vi "Enter_Rock_Data.vi"() -> ()   [LabVIEW 2019]
uses:
  Calibration.ctl
  <vilib>/Utility/NIReport.llb/Report Type.ctl
  <vilib>/addons/database/Connection.llb/DB Tools Open Connec (Path).vi
  <vilib>/addons/_office/word.llb/Word Find & Replace (str).vi
  <vilib>/addons/database/_DB Variant To Data/Database Variant To Data.xnode
  <vilib>/Utility/NIReport.llb/NI_report.lvclass
  <vilib>/addons/database/NI_Database_API.lvlib
  TEST.lvclass
  <vilib>/Utility/NIReport.llb/NI_ReportGenerationCore.lvlib
  <vilib>/addons/_office/NI_ReportGenerationToolkit.lvlib
  <vilib>/Utility/NIReport.llb/Word/NI_Word.lvclass
panel:
  in  "校准日期":timestamp format="%<%Y/%m/%d>T"
  in  "生产日期":timestamp format="%<%Y/%m/%d>T"
  in  "批号":string
  out "下沉位置":string[](array[string])
  out "误差%":string[](array[string])
  out "最大偏差":string[](array[string])
  out "测试力标准值":string[](array[string])
  in  "data":sgl[][](array[numeric]) format="%#.2g"
  out "初始化成功":bool
  out "error out":errorcluster
  in  "init":bool
  in  "NAME":string
  out "HS2":string[](array[string])
  out "CFXWC":string[](array[string])
  out "HAWC":string[](array[string])
  out "允许误差%":string[](array[string])
  out "试验力N(kg)":string[](array[string])
  out "执行状态":bool
  out "数据写入成功":bool
  in  "print_calibration":bool
  in  "print_data":bool
  in  "核验员":string
  in  "tsd":sgl[](array[numeric])=[1.0, 1.0, 1.0, 1.0] format="%#.2g"
  in  "停止":bool
  in  "write":bool
  in  "clear":bool
  in  "TEMP":string
  in  "TSN":string
  in  "MODE":string
  out "REP":sgl[](array[numeric]) format="%#.2g"
  out "HV":sgl[](array[numeric]) format="%#.2g"
  out "AVG":sgl[](array[numeric]) format="%#.2g"
  in  "TV":sgl[][](array[numeric]) format="%#.2g"
  in  "HS":sgl[](array[numeric])=[0.0, 0.0, 0.0, 0.0, 0.0] format="%#.2g"
  in  "HN":string[](array[string])
  out "Test":sgl[][](array[numeric]) format="%#.2g"
  in  "DIN":string
  out "Inacc":sgl[](array[numeric]) format="%#.2g"
  out "Dev":sgl[](array[numeric]) format="%#.2g"
  # "产品名称(首填)："
  # "型号："
  # "制造编号："
  # "温度："
  # "℃"
  # "试验力测试"
  # "2"
  # "3"
  # "1"
  # "±"
  # "±"
  # "±"
  # "±"
  # "硬度测试"
  # "金刚石压头编号："
  # "测试值"
  # "硬度块\n标准值"
  # "硬度块\n  编号"
  # "硬度值"
  # "重复性"
  # "平均值"
  # "1"
  # "2"
  # "4"
  # "5"
  # "3"
  # "实际误差"
  # "允许误差"
  # "实际误差"
  # "允许误差"
  # "±1.0"
  # "1.0RA"
  # "RA"
  # "±1.5"
  # "1.5RB"
  # "RB"
  # "±1.5"
  # "1.5RC"
  # "RC"
  # "±1.2"
  # "1.2RC"
  # "RC"
  # "±1.0"
  # "1.2RC"
  # "RC"
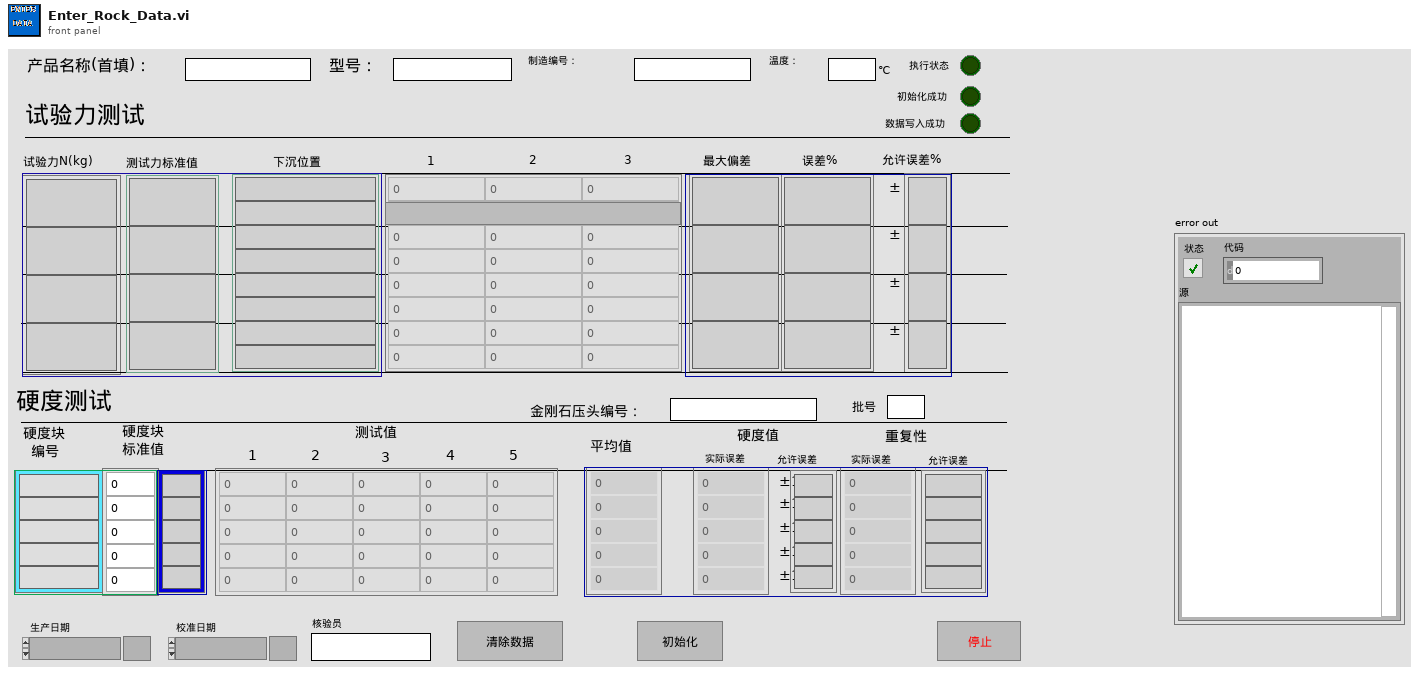
[diagram p1: front panel]
types:
  T1 = enum8{"Enabled", "Disabled", "Disabled and Grayed Out"}
  T2 = enum16{"open", "replace", "create", "open or create", "replace or create", "replace or create with confirmation"}
  T3 = typedef "TEST.lvclass/Calibration.ctl" = cluster{"NAM":string, "MODE":string, "TSN":string, "TDN":string, "DIN":string, "PROD":string, "CALD":string, "REV":string}
  T4 = typedef "NI_ReportGenerationCore.lvlib/Report Type.ctl" = enum16{"HTML", "Word", "Excel"}
  T5 = enum16{"maximized", "minimized", "normal", "no change"}
  T6 = typedef "NI_Database_API.lvlib/Conn ObjectReference.ctl" = refnum<k1>
  T7 = typedef "NI_Database_API.lvlib/DB Tools DataTypes.ctl" = enum16{"String", "Long (I32)", "Single (SGL)", "Double (DBL)", "Date/Time", "Binary"}
  T8 = cluster{"name":string, "database data type":T7, "defined size":i32}[]
  T9 = cluster{"name":string, "database data type":T7, "defined size":i32, bool}
  T10 = typedef "TEST.lvclass/Test_data.ctl" = cluster{"MODE":string, "TSN":string, "Temp":string, "Test_load_row1":T11, "Test_load_row2":T11, "Test_load_row3":T11, "Test_load_row4":T11, "DIN":string, "Hardness_test_row1":T12, "Hardness_test_row2":T12, "Hardness_test_row3":T12, "Hardness_test_row4":T12, "Hardness_test_row5":T12}
  T11 = typedef "TEST.lvclass/Test_load.ctl" = cluster{"TEST1":sgl, "TEST2":sgl, "TEST3":sgl, "DEV":sgl, "INACC":sgl}
  T12 = typedef "TEST.lvclass/Hardness_test.ctl" = cluster{"HN":string, "HS":sgl, "TV1":sgl, "TV2":sgl, "TV3":sgl, "TV4":sgl, "TV5":sgl, "AVG":sgl, "HV":sgl, "REP":sgl}
  T13 = typedef "TEST.lvclass/Cluster67.ctl" = cluster{"MOD":string, "TSN":string, "Temp":string, "TEST1":sgl, "TEST2":sgl, "TEST3":sgl, "DEV":sgl, "INACC":sgl, "TEST1":sgl, "TEST2":sgl, "TEST3":sgl, "DEV":sgl, "INACC":sgl, "TEST1":sgl, "TEST2":sgl, "TEST3":sgl, "DEV":sgl, "INACC":sgl, "TEST1":sgl, "TEST2":sgl, "TEST3":sgl, "DEV":sgl, "INACC":sgl, "DIN":string, "HN":string, "HS":sgl, "TV1":sgl, "TV2":sgl, "TV3":sgl, "TV4":sgl, "TV5":sgl, "AVG":sgl, "HV":sgl, "REP":sgl, "HN":string, "HS":sgl, "TV1":sgl, "TV2":sgl, "TV3":sgl, "TV4":sgl, "TV5":sgl, "AVG":sgl, "HV":sgl, "REP":sgl, "HN":string, "HS":sgl, "TV1":sgl, "TV2":sgl, "TV3":sgl, "TV4":sgl, "TV5":sgl, "AVG":sgl, "HV":sgl, "REP":sgl, "HN":string, "HS":sgl, "TV1":sgl, "TV2":sgl, "TV3":sgl, "TV4":sgl, "TV5":sgl, "AVG":sgl, "HV":sgl, "REP":sgl, "HN":string, "HS":sgl, "TV1":sgl, "TV2":sgl, "TV3":sgl, "TV4":sgl, "TV5":sgl, "AVG":sgl, "HV":sgl, "REP":sgl, "NAM":string, "TDN":string, "PROD":string, "CALD":string, "REV":string}
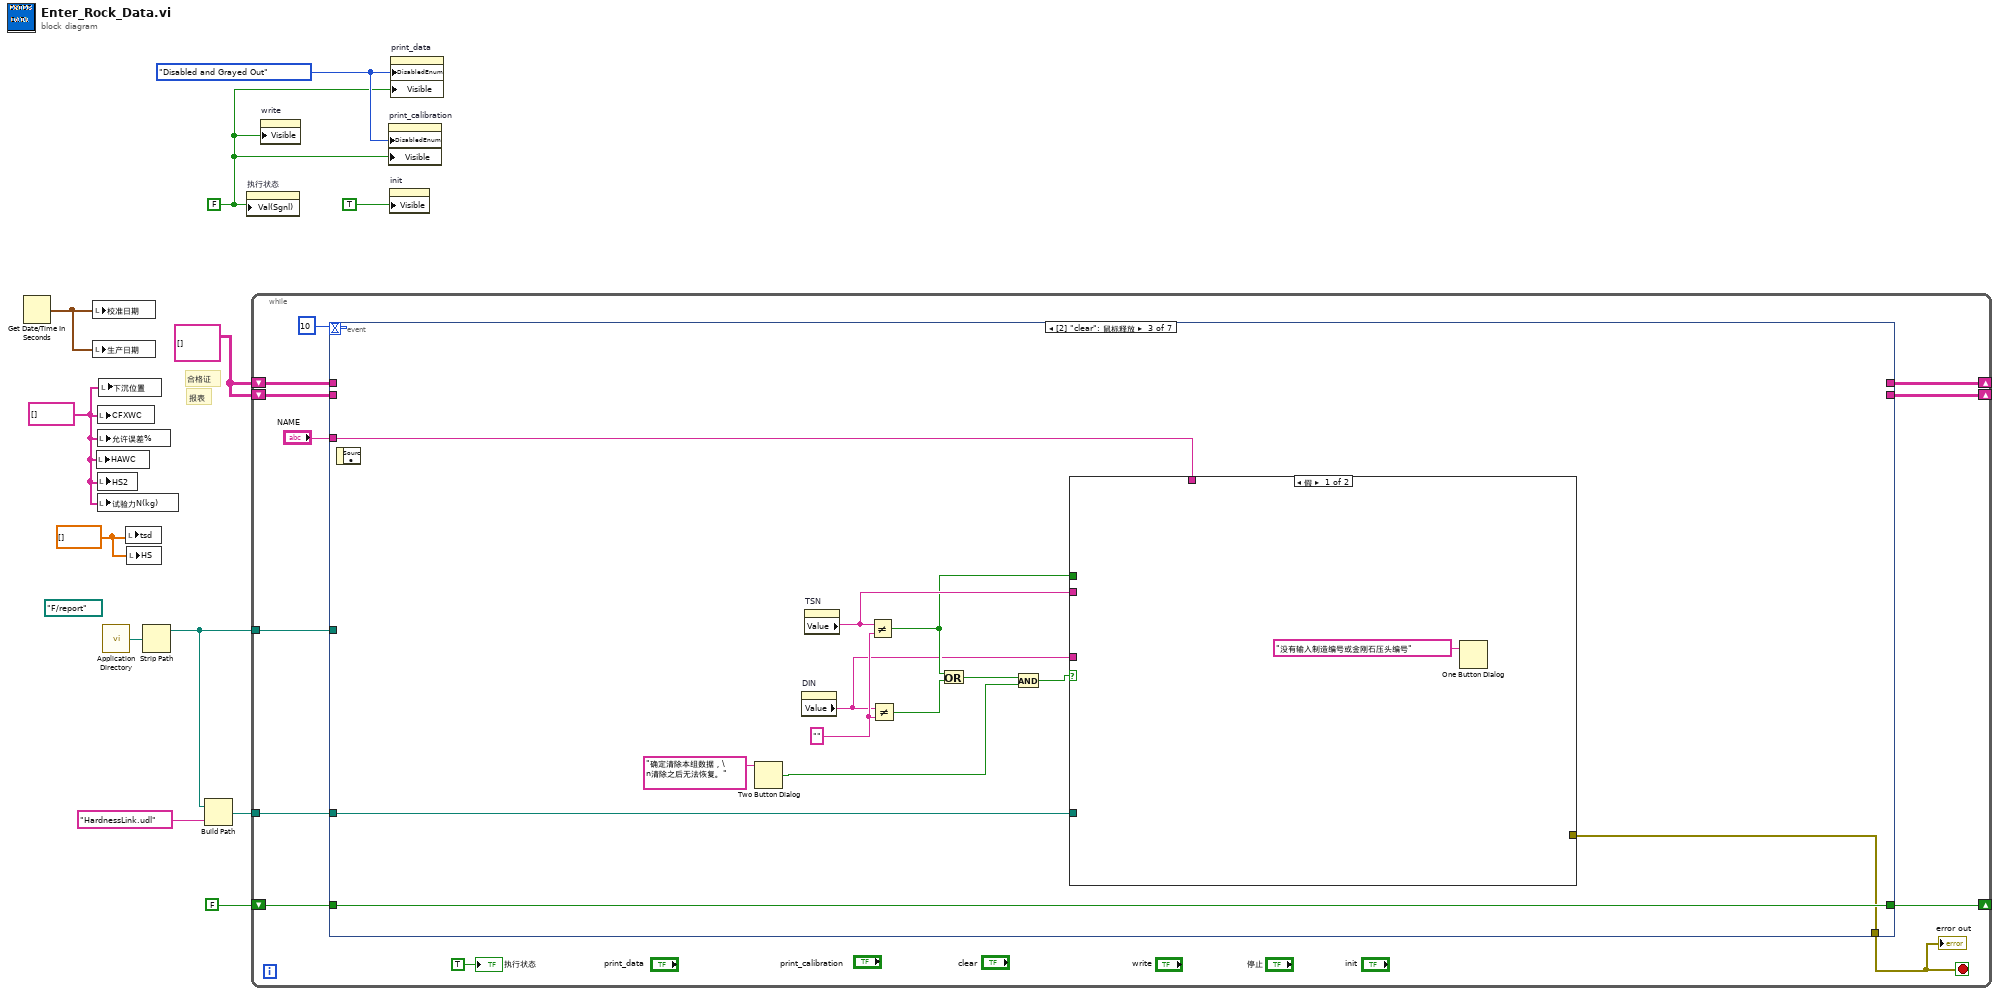
[diagram p0: block diagram]
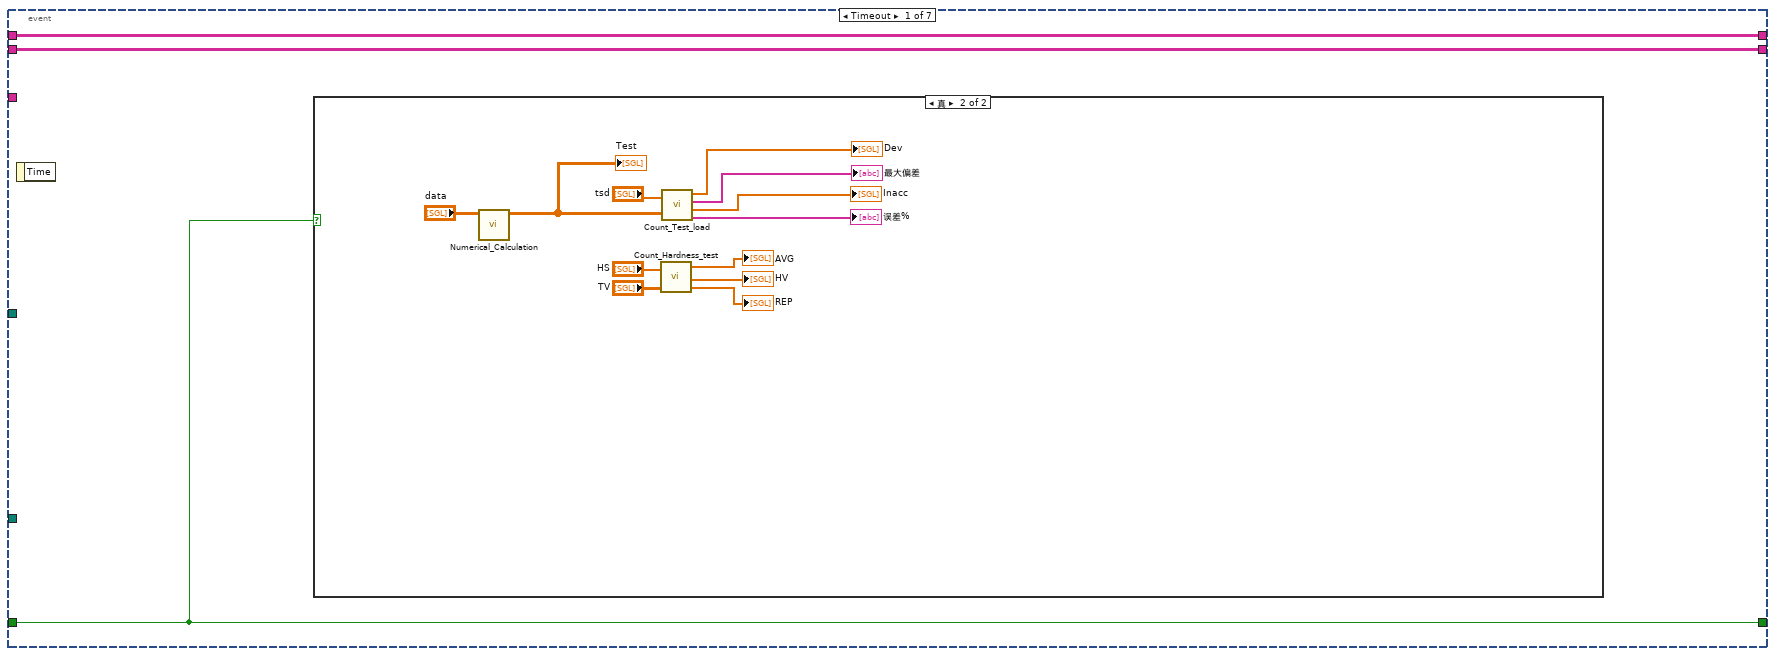
[diagram p2: hidden frame]
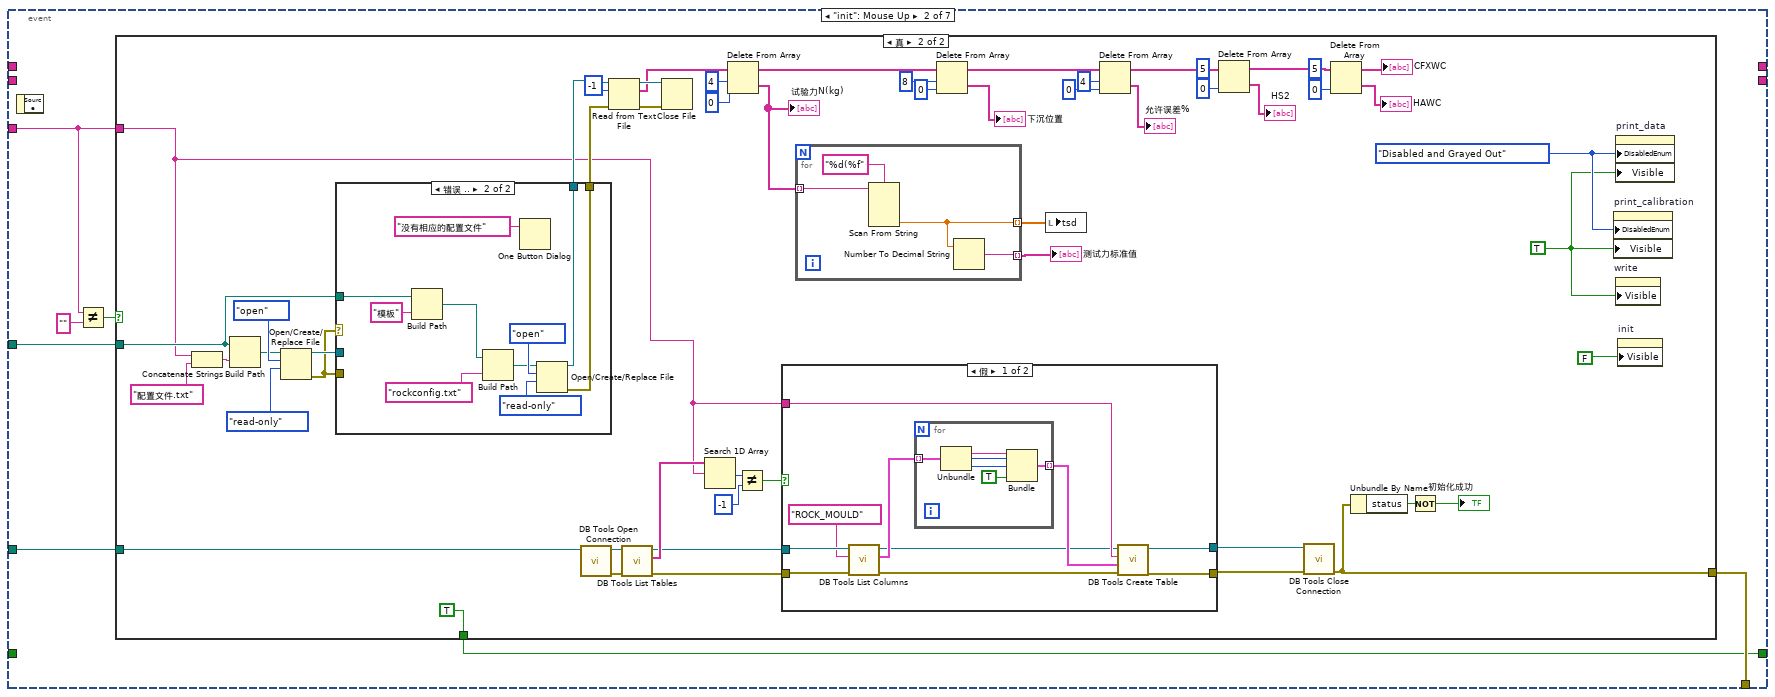
[diagram p4: hidden frame]
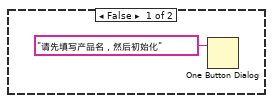
[diagram p5: hidden frame]
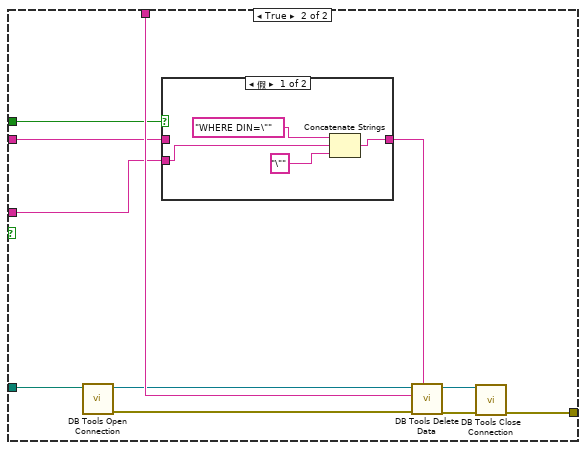
[diagram p8: hidden frame]
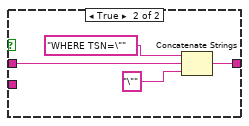
[diagram p9: hidden frame]
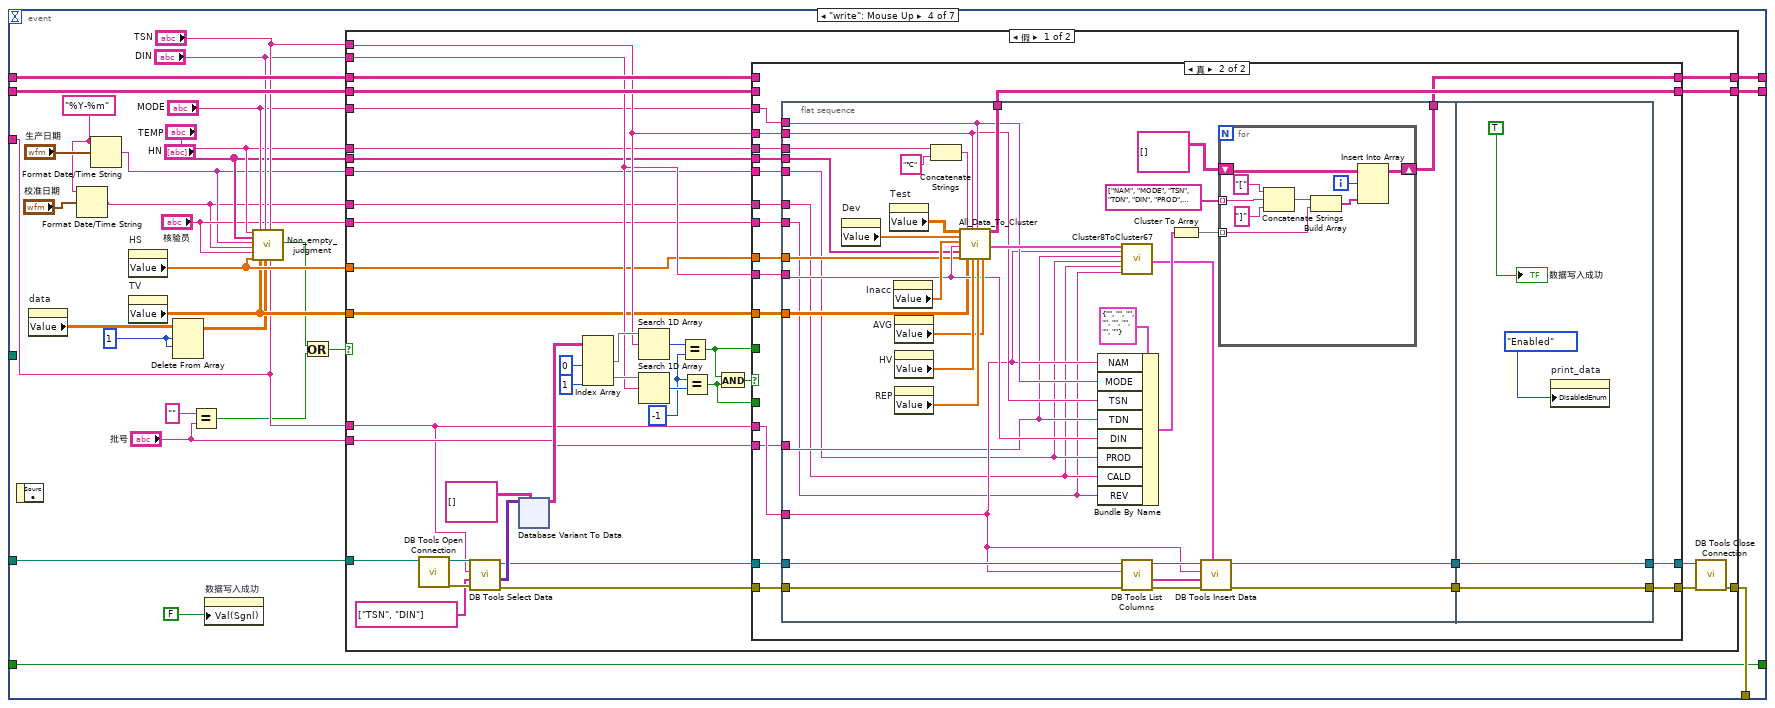
[diagram p10: hidden frame]
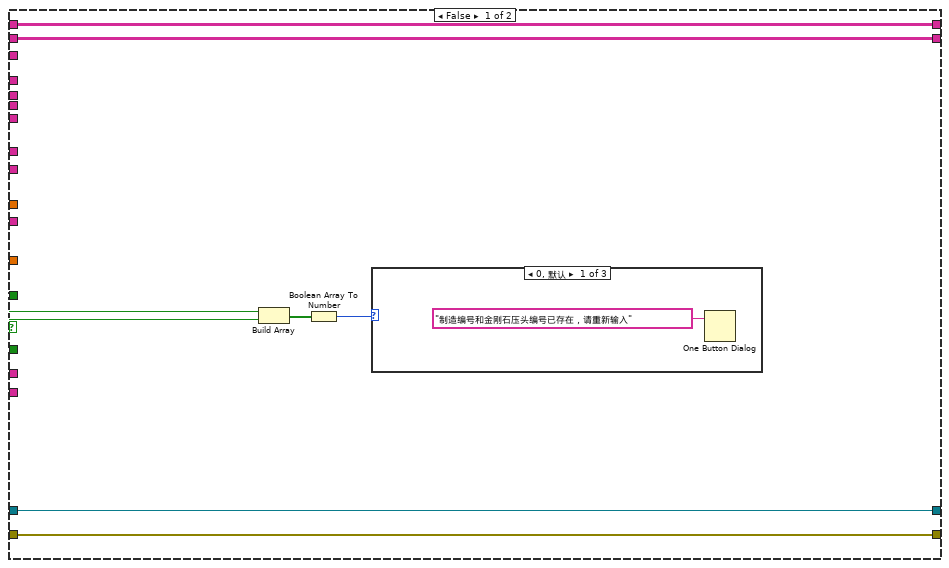
[diagram p11: hidden frame]
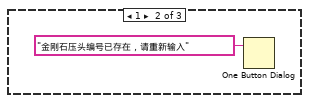
[diagram p12: hidden frame]
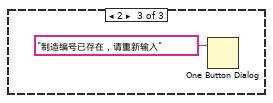
[diagram p13: hidden frame]
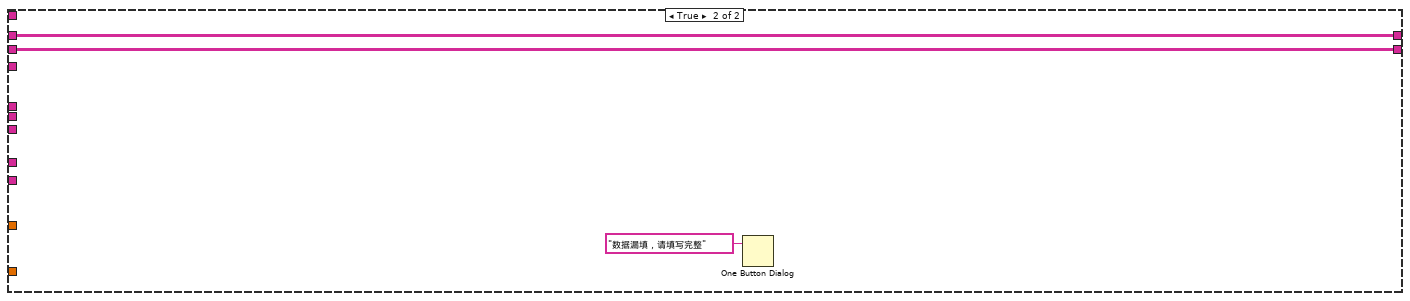
[diagram p14: hidden frame]
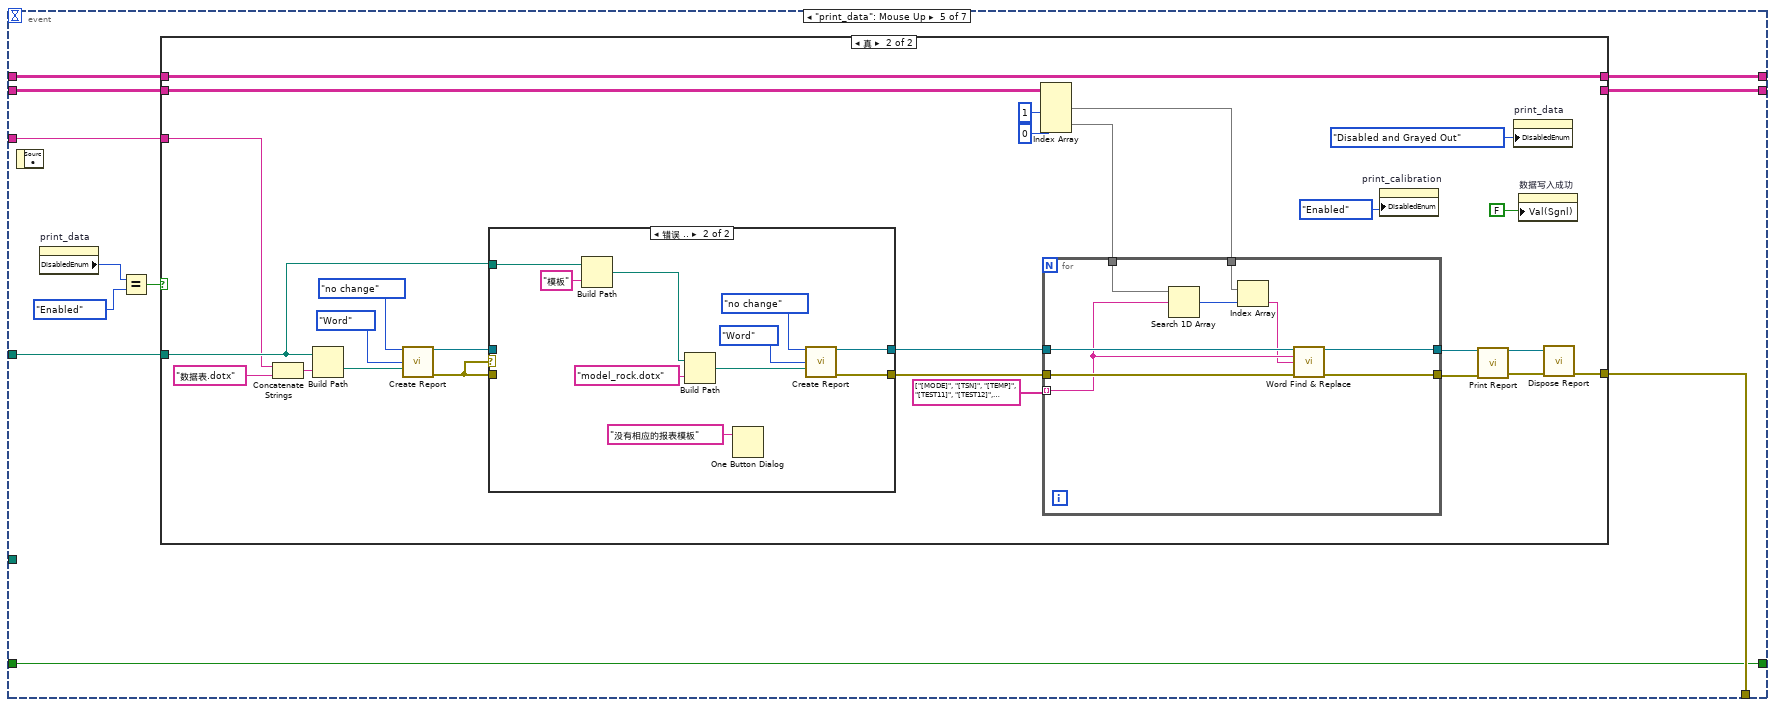
[diagram p15: hidden frame]
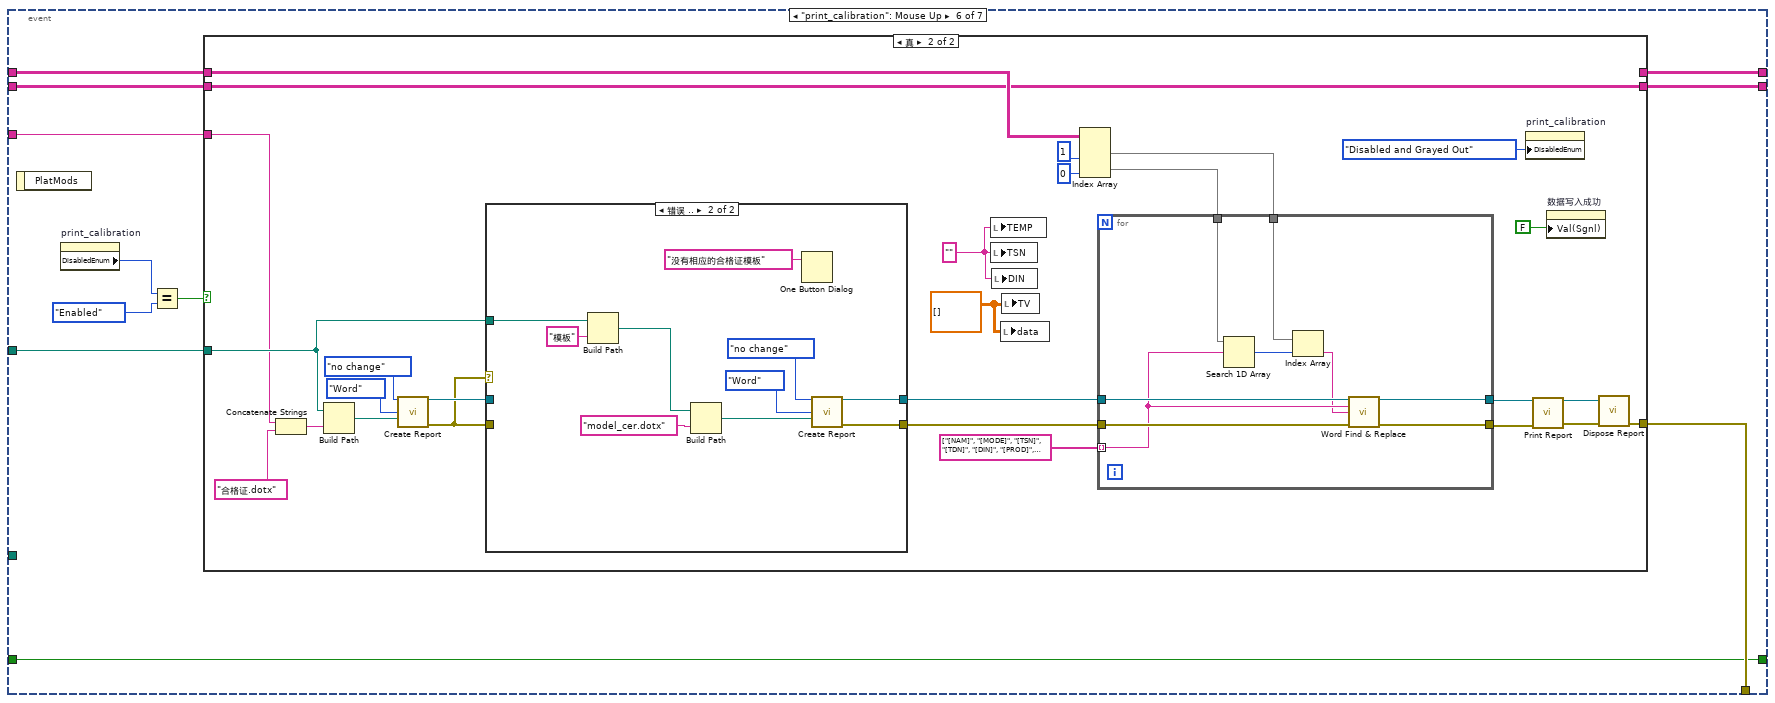
[diagram p18: hidden frame]
diagram:
  w9 = sgl[] []
  w7 = string[] []
  (unwired) path "F:/report" ("data__in")
  w8 = FALSE
  w12 = T1."Disabled and Grayed Out" ("禁用")
  w11 = string[][] []
  # "报表"
  # "合格证"
  n1 = Get Date/Time In Seconds() -> (seconds since 1Jan1904=w1:timestamp)
  n2 = local write "校准日期"(w1) -> ()
  n3 = local write "生产日期"(w1) -> ()
  n4 = local write "HAWC"(w7) -> ()
  n5 = local write "CFXWC"(w7) -> ()
  n6 = local write "允许误差%"(w7) -> ()
  n7 = local write "HS2"(w7) -> ()
  n8 = local write "试验力N(kg)"(w7) -> ()
  n9 = local write "下沉位置"(w7) -> ()
  n10 = call <vilib>:"Application Directory.vi"() -> ("Application Directory"=w5:path)
  n11 = local write "tsd"(w9) -> ()
  n12 = local write "HS"(w9) -> ()
  n13 = Strip Path(path=w5) -> (stripped path=w2:path)  [unwired: 1 out]
  n14 = Build Path(base path=w2, name or relative path="HardnessLink.udl" ("名称或相对路径")) -> (appended path=w3:path)
  n15 = property on="执行状态" class="Bool (严格)"("Val(Sgnl)"=w8) -> ()  [unwired: 2 in, 2 out]
  n16 = while {
    shift-right: [w23] -> _
    shift-left: w11 -> [w22]
    shift-right: [w20] -> _
    shift-left: w11 -> [w19]
    tunnel: w2 -> [w14]
    shift-right: [w16] -> _
    shift-left: FALSE -> [w15]
    tunnel: w3 -> [w13]
    stop <- w17 stop-if-true
    n17 = event shown="[2] \"clear\": 鼠标释放" {
      selector: _ -> [_ _ _ _ _ _ _]
      dyn-events: _ -> [_ _ _ _ _ _ _]
      timeout: 10 -> [_ _ _ _ _ _ _]
      tunnel: [_ w45 w146 w195 w375 w435 errorcluster {"status"=TRUE, "code"=0, "source"=""} ("error out")] -> w17
      tunnel: [w27 _ _ w199 w368 w430 _] -> w23
      tunnel: w22 -> [w27 _ _ w196 w371 w429 _]
      tunnel: [w26 _ _ w198 w370 w428 _] -> w20
      tunnel: w19 -> [w26 _ _ w197 w369 w431 _]
      tunnel: "NAME" -> [_ w44 w147 w186 w373 w432 _]
      tunnel: w14 -> [_ w46 _ _ w374 w434 _]
      tunnel: [w25 w41 w149 w185 w372 w433 FALSE] -> w16
      tunnel: w15 -> [w25 _ w149 w185 w372 w433 _]
      tunnel: w13 -> [_ w40 w148 w179 _ _ _]
      event Timeout {
        n18 = event-data() -> ()  [unwired: 1 in, 1 out]
        n19 = case shown="真" w25 {
          frame False {
          }
          frame True {
            n20 = call "Numerical_Calculation.vi"("Nums"="data") -> ("Calculation"=w30:sgl[][])  [unwired: 10 in]
            "Test" <- w30
            n21 = call "Count_Hardness_test.vi"("HS"="HS", "TV"="TV") -> ("AVG"=→"AVG":sgl[], "HV"=→"HV":sgl[], "REP"=→"REP":sgl[])
            n22 = call "Count_Test_load.vi"("tsd"="tsd", "Test"=w30) -> ("dev"=→"Dev":sgl[], "devs"=→"最大偏差":string[], "inacc"=→"Inacc":sgl[], "inaccs"=→"误差%":string[])
          }
        }
      }
      event "init": Mouse Up {
        n23 = event-data() -> ()  [unwired: 1 in, 1 out]
        n24 = Not Equal?(x=w44, y="" ("NAME")) -> (x != y?=w42:bool)
        n25 = case shown="真" w42 {
          tunnel: w46 -> [_ w65]
          tunnel: [_ w64] -> w45
          tunnel: w44 -> [_ w48]
          tunnel: [_ TRUE] -> w41
          tunnel: w40 -> [_ w49]
          frame False {
            n26 = One Button Dialog(message="请先填写产品名，然后初始化" ("消息")) -> ()  [unwired: 1 in, 1 out]
          }
          frame True {
            w91 = T1."Disabled and Grayed Out" ("禁用")
            w90 = TRUE ("可见")
            n27 = Concatenate Strings(w48, "配置文件.txt" ("名称或相对路径")) -> (w70:string)
            n28 = Build Path(base path=w65, name or relative path=w70) -> (appended path=w84:path)
            n29 = Open/Create/Replace File(file path (use dialog)=w84, operation (0:open)=T2."open" ("操作(0:open)"), access (0:read/write)=enum16{"read/write", "read-only", "write-only"}."read-only" ("权限(0:read/write)")) -> (refnum out=w68:refnum<file>, error out=w66:errorcluster)  [unwired: 3 in, 1 out]
            n30 = case shown="错误 .." w66 {
              tunnel: [w108 w118] -> w69
              tunnel: w68 -> [w108 _]
              tunnel: [w107 w117] -> w67
              tunnel: w66 -> [w107 _]
              tunnel: w65 -> [_ w112]
              frame No Error {
              }
              frame Error {
                n31 = Build Path(base path=w112, name or relative path="模板" ("名称或相对路径")) -> (appended path=w110:path)
                n32 = Build Path(base path=w110, name or relative path="rockconfig.txt") -> (appended path=w114:path)
                n33 = One Button Dialog(message="没有相应的配置文件" ("消息")) -> ()  [unwired: 1 in, 1 out]
                n34 = Open/Create/Replace File(file path (use dialog)=w114, operation (0:open)=T2."open" ("操作(0:open)"), access (0:read/write)=enum16{"read/write", "read-only", "write-only"}."read-only" ("权限(0:read/write)")) -> (refnum out=w118:refnum<file>, error out=w117:errorcluster)  [unwired: 3 in, 1 out]
              }
            }
            n35 = call-poly <vilib>:"DB Tools Open Connection.vi"("connection information"=w49) -> ("error out"=w101:errorcluster, "connection reference"=w102:T6)  [unwired: 7 in]
            n36 = Read from Text File(file (use dialog)=w69, count=-1 ("计数"), error in=w67) -> (refnum out=w86:refnum<file>, text=w83:string[], error out=w87:errorcluster)  [unwired: 1 in, 1 out]
            n37 = call <vilib>:"DB Tools List Tables.vi"("error in (no error)"=w101, "connection reference"=w102) -> ("error out"=w95:errorcluster, "tables"=w100:string[], "connection reference out"=w96:T6)  [unwired: 3 in]
            n38 = Close File(refnum=w86, error in=w87) -> ()  [unwired: 2 out]
            n39 = Search 1D Array(1D array=w100, element=w48) -> (index of element=w99:i32)  [unwired: 1 in]
            n40 = Delete From Array(array=w83, length=4 ("长度"), index=0 ("索引")) -> (deleted portion=w60:string[], array with subset deleted=w80:string[])
            "试验力N(kg)" <- w60
            n41 = Not Equal?(x=w99, y=-1) -> (x != y?=w97:bool)
            n42 = case shown="假" w97 {
              tunnel: [w120 w136] -> w93
              tunnel: w96 -> [w128 w136]
              tunnel: w95 -> [w127 w135]
              tunnel: [w119 w135] -> w94
              tunnel: w48 -> [w123 _]
              frame False {
                n43 = call <vilib>:"DB Tools List Columns.vi"("error in (no error)"=w127, "table"="ROCK_MOULD", "connection reference"=w128) -> ("error out"=w121:errorcluster, "column information"=w125:T8, "connection reference out"=w122:T6)  [unwired: 1 in, 1 out]
                n44 = for {
                  tunnel: w125 -> [w134] mode=indexing
                  tunnel: [w129] -> w124 mode=indexing
                  n45 = Unbundle(w134) -> ("name"=w133:string, "database data type"=w132:T7, "defined size"=w131:i32)
                  n46 = Bundle("name"=w133, "database data type"=w132, "defined size"=w131, TRUE) -> (w129:T9)  [unwired: 1 in]
                }
                n47 = call <vilib>:"DB Tools Create Table.vi"("error in (no error)"=w121, "column information"=w124, "table"=w123, "connection reference"=w122) -> ("error out"=w119:errorcluster, "connection reference out"=w120:T6)  [unwired: 4 in]
              }
              frame True {
              }
            }
            n48 = for {
              tunnel: w60 -> [w105] mode=indexing
              tunnel: [w104] -> w61 mode=indexing
              tunnel: [w103] -> w55 mode=indexing
              n49 = Scan From String(format string="%d(%f" ("格式字符串"), input string=w105) -> (output 2=w104:dbl)  [unwired: 5 in, 3 out]
              n50 = Number To Decimal String(number=w104) -> (decimal integer string=w103:string)  [unwired: 1 in]
            }
            "测试力标准值" <- w55
            n51 = Delete From Array(array=w80, length=8 ("长度"), index=0 ("索引")) -> (deleted portion=→"下沉位置":string[], array with subset deleted=w54:string[])
            n52 = local write "tsd"(w61) -> ()
            n53 = Delete From Array(array=w54, length=4 ("长度"), index=0 ("索引")) -> (deleted portion=→"允许误差%":string[], array with subset deleted=w77:string[])
            n54 = Delete From Array(array=w77, length=5 ("长度"), index=0 ("索引")) -> (deleted portion=→"HS2":string[], array with subset deleted=w74:string[])
            n55 = call <vilib>:"DB Tools Close Connection.vi"("error in (no error)"=w94, "connection reference"=w93) -> ("error out"=w64:errorcluster)  [unwired: 5 in]
            n56 = Delete From Array(array=w74, length=5 ("长度"), index=0 ("索引")) -> (deleted portion=→"HAWC":string[], array with subset deleted=→"CFXWC":string[])
            n57 = Unbundle By Name(w64) -> ("status"=w63:bool)
            n58 = Not(x=w63) -> (.not. x?=→"初始化成功":bool)
            n59 = property on="print_calibration" class="Bool (严格)"("DisabledEnum"=w91, "Visible"=w90) -> ()  [unwired: 2 in, 2 out]
            n60 = property on="print_data" class="Bool (严格)"("DisabledEnum"=w91, "Visible"=w90) -> ()  [unwired: 2 in, 2 out]
            n61 = property on="write" class="Bool (严格)"("Visible"=w90) -> ()  [unwired: 2 in, 2 out]
            n62 = property on="init" class="Bool (严格)"("Visible"=FALSE ("可见")) -> ()  [unwired: 2 in, 2 out]
          }
        }
      }
      event "clear": Mouse Up {
        w145 = ""
        n63 = event-data() -> ()  [unwired: 1 in, 1 out]
        n64 = Two Button Dialog(message="确定清除本组数据，\n清除之后无法恢复。" ("消息")) -> (T button?=w138:bool)  [unwired: 2 in]
        n65 = property on="DIN" class="Str"() -> ("Value"=w141:string)  [unwired: 2 in, 2 out]
        n66 = property on="TSN" class="Str"() -> ("Value"=w143:string)  [unwired: 2 in, 2 out]
        n67 = Not Equal?(x=w143, y=w145) -> (x != y?=w142:bool)
        n68 = Not Equal?(x=w141, y=w145) -> (x != y?=w144:bool)
        n69 = Or(x=w142, y=w144) -> (x .or. y?=w139:bool)
        n70 = And(x=w139, y=w138) -> (x .and. y?=w137:bool)
        n71 = case shown="假" w137 {
          tunnel: w148 -> [_ w161]
          tunnel: w147 -> [_ w160]
          tunnel: [_ w159] -> w146
          tunnel: w143 -> [_ w153]
          tunnel: w142 -> [_ w152]
          tunnel: w141 -> [_ w151]
          frame False {
            n72 = One Button Dialog(message="没有输入制造编号或金刚石压头编号" ("消息")) -> ()  [unwired: 1 in, 1 out]
          }
          frame True {
            n73 = call-poly <vilib>:"DB Tools Open Connection.vi"("connection information"=w161) -> ("error out"=w157:errorcluster, "connection reference"=w158:T6)  [unwired: 7 in]
            n74 = case shown="假" w152 {
              tunnel: [w163 w167] -> w154
              tunnel: w153 -> [_ w166]
              tunnel: w151 -> [w162 _]
              frame False {
                n75 = Concatenate Strings("WHERE DIN=\"", w162, "\"" ("字符串")) -> (w163:string)
              }
              frame True {
                n76 = Concatenate Strings("WHERE TSN=\"", w166, "\"" ("字符串")) -> (w167:string)
              }
            }
            n77 = call <vilib>:"DB Tools Delete Data.vi"("condition"=w154, "error in (no error)"=w157, "table"=w160, "connection reference"=w158) -> ("error out"=w156:errorcluster, "connection reference out"=w155:T6)  [unwired: 6 in]
            n78 = call <vilib>:"DB Tools Close Connection.vi"("error in (no error)"=w156, "connection reference"=w155) -> ("error out"=w159:errorcluster)  [unwired: 5 in]
          }
        }
      }
      event "write": Mouse Up {
        w171 = 1 ("长度")
        w175 = "%Y-%m" ("时间格式字符串(%c)")
        n79 = event-data() -> ()  [unwired: 1 in, 1 out]
        n80 = property on="data" class="Arr (严格)"() -> ("Value"=w173:sgl[][])  [unwired: 2 in, 2 out]
        n81 = Format Date/Time String(time format string (%c)=w175, seconds (now)="校准日期") -> (date/time string=w174:string)  [unwired: 1 in]
        n82 = Format Date/Time String(time format string (%c)=w175, seconds (now)="生产日期") -> (date/time string=w177:string)  [unwired: 1 in]
        n83 = property on="HS" class="Arr (严格)"() -> ("Value"=w188:sgl[])  [unwired: 2 in, 2 out]
        n84 = property on="TV" class="Arr (严格)"() -> ("Value"=w187:sgl[][])  [unwired: 2 in, 2 out]
        n85 = Delete From Array(array=w173, length=w171, index (row)=w171) -> (array with subset deleted=w172:sgl[][])  [unwired: 1 in, 1 out]
        n86 = Equal?(x="", y="批号") -> (x = y?=w180:bool)
        n87 = property on="数据写入成功" class="Bool (严格)"("Val(Sgnl)"=FALSE) -> ()  [unwired: 2 in, 2 out]
        n88 = call "Non_empty_judgment.vi"("TEMP"="TEMP", "HN"="HN", "生产日期"=w177, "校准日期"=w174, "核验员"="核验员", "HS"=w188, "MODE"="MODE", "TV"=w187, "DIN"="DIN", "TESTS"=w172, "TSN"="TSN", "NAME"=w186) -> ("结果"=w181:bool)  [unwired: 7 in]
        n89 = Or(x=w181, y=w180) -> (x .or. y?=w170:bool)
        n90 = case shown="假" w170 {
          tunnel: [w237 w363] -> w199
          tunnel: [w236 w364] -> w198
          tunnel: w197 -> [w221 w364]
          tunnel: w196 -> [w220 w363]
          tunnel: w179 -> [w219 _]
          tunnel: [w212 _] -> w195
          tunnel: "TSN" -> [w211 _]
          tunnel: "DIN" -> [w210 _]
          tunnel: "MODE" -> [w209 _]
          tunnel: "TEMP" -> [w208 _]
          tunnel: "HN" -> [w207 _]
          tunnel: w177 -> [w206 _]
          tunnel: w174 -> [w205 _]
          tunnel: "核验员" -> [w204 _]
          tunnel: w188 -> [w203 _]
          tunnel: w187 -> [w202 _]
          tunnel: w186 -> [w200 _]
          tunnel: "批号" -> [w201 _]
          frame False {
            w223 = -1
            n91 = call-poly <vilib>:"DB Tools Open Connection.vi"("connection information"=w219) -> ("error out"=w234:errorcluster, "connection reference"=w235:T6)  [unwired: 7 in]
            n92 = call <vilib>:"DB Tools Select Data.vi"("error in (no error)"=w234, "columns"=string[] ["TSN", "DIN"], "table"=w200, "connection reference"=w235) -> ("error out"=w215:errorcluster, "data"=w232:variant[][], "connection reference out"=w216:T6)  [unwired: 2 in]
            n93 = xnode "Database Variant To Data"("database variant"=w232, "type"=string[][] []) -> ("data"=w230:string[][])  [unwired: 1 in, 1 out]
            n94 = Index Array(array=w230, index (col) #1=0 ("禁用的索引 (列)"), index (col) #2=1 ("索引 (列)")) -> (element #1=w227:string[], element #2=w226:string[])  [unwired: 2 in]
            n95 = Search 1D Array(1D array=w227, element=w211) -> (index of element=w225:i32)  [unwired: 1 in]
            n96 = Search 1D Array(1D array=w226, element=w210) -> (index of element=w224:i32)  [unwired: 1 in]
            n97 = Equal?(x=w225, y=w223) -> (x = y?=w218:bool)
            n98 = Equal?(x=w223, y=w224) -> (x = y?=w217:bool)
            n99 = And(x=w218, y=w217) -> (x .and. y?=w222:bool)
            n100 = case shown="真" w222 {
              tunnel: [w244 w268] -> w237
              tunnel: [w245 w267] -> w236
              tunnel: w211 -> [_ w266]
              tunnel: w210 -> [_ w265]
              tunnel: w221 -> [w245 _]
              tunnel: w220 -> [w244 _]
              tunnel: w200 -> [_ w264]
              tunnel: w218 -> [w242 _]
              tunnel: w217 -> [w243 _]
              tunnel: w216 -> [w239 w263]
              tunnel: w215 -> [w238 w262]
              tunnel: [w239 w260] -> w214
              tunnel: [w238 w258] -> w213
              tunnel: w209 -> [_ w257]
              tunnel: w208 -> [_ w256]
              tunnel: w207 -> [_ w255]
              tunnel: w206 -> [_ w254]
              tunnel: w203 -> [_ w253]
              tunnel: w202 -> [_ w252]
              tunnel: w205 -> [_ w251]
              tunnel: w204 -> [_ w250]
              tunnel: w201 -> [_ w249]
              frame False {
                n101 = Build Array(w242, w243) -> (w241:bool[])
                n102 = Boolean Array To Number(Boolean array=w241) -> (number=w240:u32)
                n103 = case shown="0, 默认" w240 {
                  frame 0, Default {
                    n104 = One Button Dialog(message="制造编号和金刚石压头编号已存在，请重新输入" ("消息")) -> ()  [unwired: 1 in, 1 out]
                  }
                  frame 1 {
                    n105 = One Button Dialog(message="金刚石压头编号已存在，请重新输入" ("消息")) -> ()  [unwired: 1 in, 1 out]
                  }
                  frame 2 {
                    n106 = One Button Dialog(message="制造编号已存在，请重新输入" ("消息")) -> ()  [unwired: 1 in, 1 out]
                  }
                }
              }
              frame True {
                n107 = flat-sequence {
                  tunnel: [w291] -> w268
                  tunnel: [w288] -> w267
                  tunnel: w266 -> [w278]
                  tunnel: w265 -> [w286]
                  tunnel: w264 -> [w273]
                  tunnel: w263 -> [w277]
                  tunnel: w262 -> [w276]
                  tunnel: [w285] -> w261
                  tunnel: [w284] -> w259
                  tunnel: w257 -> [w279]
                  tunnel: w256 -> [w283]
                  tunnel: w255 -> [w282]
                  tunnel: w254 -> [w271]
                  tunnel: w253 -> [w281]
                  tunnel: w252 -> [w280]
                  tunnel: w251 -> [w270]
                  tunnel: w250 -> [w269]
                  tunnel: w249 -> [w272]
                  tunnel: w261 -> [w315]
                  tunnel: [w315] -> w260
                  tunnel: w259 -> [w314]
                  tunnel: [w314] -> w258
                  frame #0 {
                    n108 = property on="Dev" class="Arr (严格)"() -> ("Value"=w300:sgl[])  [unwired: 2 in, 2 out]
                    n109 = property on="Test" class="Arr (严格)"() -> ("Value"=w301:sgl[][])  [unwired: 2 in, 2 out]
                    n110 = property on="Inacc" class="Arr (严格)"() -> ("Value"=w299:sgl[])  [unwired: 2 in, 2 out]
                    n111 = property on="AVG" class="Arr (严格)"() -> ("Value"=w296:sgl[])  [unwired: 2 in, 2 out]
                    n112 = property on="HV" class="Arr (严格)"() -> ("Value"=w298:sgl[])  [unwired: 2 in, 2 out]
                    n113 = property on="REP" class="Arr (严格)"() -> ("Value"=w297:sgl[])  [unwired: 2 in, 2 out]
                    n114 = Concatenate Strings(w283, "℃") -> (w293:string)
                    n115 = call "All_Data_To_Cluster.vi"("Test"=w301, "Dev"=w300, "Inacc"=w299, "DIN"=w286, "HN"=w282, "HS"=w281, "TEMP"=w293, "TV"=w280, "TSN"=w278, "HV"=w298, "MODE"=w279, "REP"=w297, "AVG"=w296) -> ("All_data_String"=w291:string[][], "Test_Data"=w295:T10)  [unwired: 5 in]
                    n116 = Bundle By Name(cluster=T3 {"NAM"="", "MODE"="", "TSN"="", "TDN"="", "DIN"="", "PROD"="", "CALD"="", "REV"=""} ("Cal"), "NAM"=w273, "MODE"=w279, "TSN"=w278, "TDN"=w272, "DIN"=w286, "PROD"=w271, "CALD"=w270, "REV"=w269) -> (w287:T3)
                    n117 = call "Cluster8ToCluster67.vi"("簇"=w295, "NAM"=w273, "TDN"=w272, "PROD"=w271, "CALD"=w270, "REV"=w269) -> ("输出簇"=w274:T13)  [unwired: 13 in]
                    n118 = call <vilib>:"DB Tools List Columns.vi"("error in (no error)"=w276, "table"=w273, "connection reference"=w277) -> ("error out"=w304:errorcluster, "columns"=w303:string[], "connection reference out"=w302:T6)  [unwired: 1 in, 1 out]
                    n119 = Cluster To Array(cluster=w287) -> (array=w290:string[])
                    n120 = call <vilib>:"DB Tools Insert Data.vi"("data"=w274, "error in (no error)"=w304, "columns"=w303, "table"=w273, "connection reference"=w302) -> ("error out"=w284:errorcluster, "connection reference out"=w285:T6)  [unwired: 5 in]
                    n121 = for {
                      tunnel: w290 -> [w313] mode=indexing
                      shift-right: [w311] -> w288
                      shift-left: string[][] [] -> [w312]
                      tunnel: string[] ["NAM", "MODE", "TSN", "TDN", "DIN", "PROD", "CALD", "REV"] ("columns 3") -> [w305] mode=indexing
                      i -> [w310]
                      n122 = Concatenate Strings("[" ("字符串"), w305, "]" ("字符串")) -> (w307:string)
                      n123 = Build Array(w307, w313) -> (w306:string[])
                      n124 = Insert Into Array(array=w312, index (row)=w310, new element=w306) -> (w311:string[][])  [unwired: 1 in]
                    }
                  }
                  frame #1 {
                    n125 = property on="print_data" class="Bool (严格)"("DisabledEnum"=T1."Enabled" ("禁用")) -> ()  [unwired: 2 in, 2 out]
                    "数据写入成功" <- TRUE
                  }
                }
              }
            }
            n126 = call <vilib>:"DB Tools Close Connection.vi"("error in (no error)"=w213, "connection reference"=w214) -> ("error out"=w212:errorcluster)  [unwired: 5 in]
          }
          frame True {
            n127 = One Button Dialog(message="数据漏填，请填写完整" ("消息")) -> ()  [unwired: 1 in, 1 out]
          }
        }
      }
      event "print_data": Mouse Up {
        n128 = event-data() -> ()  [unwired: 1 in, 1 out]
        n129 = property on="print_data" class="Bool (严格)"() -> ("DisabledEnum"=w366:T1)  [unwired: 2 in, 2 out]
        n130 = Equal?(x=w366, y=T1."Enabled" ("禁用")) -> (x = y?=w367:bool)
        n131 = case shown="真" w367 {
          tunnel: [_ w392] -> w375
          tunnel: w374 -> [_ w387]
          tunnel: w373 -> [_ w386]
          tunnel: w371 -> [w376 w384]
          tunnel: [w377 w379] -> w370
          tunnel: w369 -> [w377 w379]
          tunnel: [w376 _] -> w368
          frame False {
          }
          frame True {
            n132 = Concatenate Strings(w386, "数据表.dotx" ("字符串")) -> (w393:string)
            n133 = Build Path(base path=w387, name or relative path=w393) -> (appended path=w395:path)
            n134 = call <vilib>:"Create Report.vi"("window state (normal)"=T5."no change", "report type"=Report_Type."Word", "template (empty)"=w395) -> ("report out"=w388:refnum<class "NI_report.lvclass">, "error out"=w391:errorcluster)  [unwired: 11 in]
            n135 = case shown="错误 .." w391 {
              tunnel: w391 -> [w405 _]
              tunnel: [w405 w413] -> w390
              tunnel: [w404 w412] -> w389
              tunnel: w388 -> [w404 _]
              tunnel: w387 -> [_ w409]
              frame No Error {
              }
              frame Error {
                n136 = Build Path(base path=w409, name or relative path="模板" ("名称或相对路径")) -> (appended path=w407:path)
                n137 = Build Path(base path=w407, name or relative path="model_rock.dotx") -> (appended path=w410:path)
                n138 = One Button Dialog(message="没有相应的报表模板" ("消息")) -> ()  [unwired: 1 in, 1 out]
                n139 = call <vilib>:"Create Report.vi"("window state (normal)"=T5."no change", "report type"=Report_Type."Word", "template (empty)"=w410) -> ("report out"=w412:refnum<class "NI_report.lvclass">, "error out"=w413:errorcluster)  [unwired: 11 in]
              }
            }
            n140 = Index Array(array=w384, index (col) #1=1 ("禁用的索引 (列)"), index (col) #2=0 ("索引 (列)")) -> (element #1=w380:string[], element #2=w381:string[])  [unwired: 2 in]
            n141 = for {
              tunnel: string[] ["[MODE]", "[TSN]", "[TEMP]", "[TEST11]", "[TEST12]", "[TEST13]", "[DEV1]", "[INACC1]", "[TEST21]", "[TEST22]", "[TEST23]", "[DEV2]", "[INACC2]", "[TEST31]", "[TEST32]", "[TEST33]", "[DEV3]", "[INACC3]", "[TEST41]", "[TEST42]", "[TEST43]", "[DEV4]", "[INACC4]", "[DIN]", "[HN1]", "[HS1]", "[TV11]", "[TV12]", "[TV13]", "[TV14]", "[TV15]", "[AVG1]", "[HV1]", "[REP1]", "[HN2]", "[HS2]", "[TV21]", "[TV22]", "[TV23]", "[TV24]", "[TV25]", "[AVG2]", "[HV2]", "[REP2]", "[HN3]", "[HS3]", "[TV31]", "[TV32]", "[TV33]", "[TV34]", "[TV35]", "[AVG3]", "[HV3]", "[REP3]", "[HN4]", "[HS4]", "[TV41]", "[TV42]", "[TV43]", "[TV44]", "[TV45]", "[AVG4]", "[HV4]", "[REP4]", "[HN5]", "[HS5]", "[TV51]", "[TV52]", "[TV53]", "[TV54]", "[TV55]", "[AVG5]", "[HV5]", "[REP5]"] ("待写入项") -> [w420] mode=indexing
              tunnel: w389 -> [w424]
              tunnel: [w422] -> w400
              tunnel: w390 -> [w423]
              tunnel: [w421] -> w401
              tunnel: w381 -> [w416]
              tunnel: w380 -> [w417]
              n142 = Search 1D Array(1D array=w416, element=w420) -> (index of element=w419:i32)  [unwired: 1 in]
              n143 = Index Array(array=w417, index=w419) -> (element=w418:string)
              n144 = call-poly <vilib>:"Word Find & Replace.vi"("report in"=w424, "find what?"=w420, "replace with"=w418, "error in (no error)"=w423) -> ("report out"=w422:refnum<class "NI_report.lvclass">, "error out"=w421:errorcluster)  [unwired: 9 in, 1 out]
            }
            n145 = property on="print_calibration" class="Bool (严格)"("DisabledEnum"=T1."Enabled" ("禁用")) -> ()  [unwired: 2 in, 2 out]
            n146 = call-dynamic "Print Report.vi"("report in"=w400, "error in (no error)"=w401) -> ("report out"=w398:refnum<class "NI_report.lvclass">, "error out"=w399:errorcluster)  [unwired: 12 in]
            n147 = property on="print_data" class="Bool (严格)"("DisabledEnum"=T1."Disabled and Grayed Out" ("禁用")) -> ()  [unwired: 2 in, 2 out]
            n148 = property on="数据写入成功" class="Bool (严格)"("Val(Sgnl)"=FALSE) -> ()  [unwired: 2 in, 2 out]
            n149 = call-dynamic "Dispose Report.vi"("report in"=w398, "error in (no error)"=w399) -> ("error out"=w392:errorcluster)  [unwired: 13 in]
          }
        }
      }
      event "print_calibration": Mouse Up {
        n150 = event-data() -> ()  [unwired: 1 in, 1 out]
        n151 = property on="print_calibration" class="Bool (严格)"() -> ("DisabledEnum"=w426:T1)  [unwired: 2 in, 2 out]
        n152 = Equal?(x=w426, y=T1."Enabled" ("禁用")) -> (x = y?=w427:bool)
        n153 = case shown="真" w427 {
          tunnel: [_ w458] -> w435
          tunnel: w434 -> [_ w448]
          tunnel: w432 -> [_ w446]
          tunnel: w431 -> [w436 w443]
          tunnel: [w437 w438] -> w430
          tunnel: w429 -> [w437 w438]
          tunnel: [w436 _] -> w428
          frame False {
          }
          frame True {
            w445 = sgl[][] []
            w444 = ""
            n154 = Concatenate Strings(w446, "合格证.dotx" ("字符串")) -> (w454:string)
            n155 = Build Path(base path=w448, name or relative path=w454) -> (appended path=w455:path)
            n156 = call <vilib>:"Create Report.vi"("window state (normal)"=T5."no change", "report type"=Report_Type."Word", "template (empty)"=w455) -> ("report out"=w451:refnum<class "NI_report.lvclass">, "error out"=w450:errorcluster)  [unwired: 11 in]
            n157 = case shown="错误 .." w450 {
              tunnel: [w466 w469] -> w452
              tunnel: w451 -> [w466 _]
              tunnel: w450 -> [w465 _]
              tunnel: [w465 w468] -> w449
              tunnel: w448 -> [_ w470]
              frame No Error {
              }
              frame Error {
                n158 = Build Path(base path=w470, name or relative path="模板" ("名称或相对路径")) -> (appended path=w471:path)
                n159 = Build Path(base path=w471, name or relative path="model_cer.dotx") -> (appended path=w473:path)
                n160 = One Button Dialog(message="没有相应的合格证模板" ("消息")) -> ()  [unwired: 1 in, 1 out]
                n161 = call <vilib>:"Create Report.vi"("window state (normal)"=T5."no change", "report type"=Report_Type."Word", "template (empty)"=w473) -> ("report out"=w469:refnum<class "NI_report.lvclass">, "error out"=w468:errorcluster)  [unwired: 11 in]
              }
            }
            n162 = local write "TEMP"(w444) -> ()
            n163 = local write "TSN"(w444) -> ()
            n164 = local write "DIN"(w444) -> ()
            n165 = local write "data"(w445) -> ()
            n166 = local write "TV"(w445) -> ()
            n167 = Index Array(array=w443, index (col) #1=1 ("禁用的索引 (列)"), index (col) #2=0 ("禁用的索引 (列)")) -> (element #1=w439:string[], element #2=w440:string[])  [unwired: 2 in]
            n168 = for {
              tunnel: string[] ["[NAM]", "[MODE]", "[TSN]", "[TDN]", "[DIN]", "[PROD]", "[CALD]", "[REV]"] ("待写入项 2") -> [w481] mode=indexing
              tunnel: w452 -> [w485]
              tunnel: [w483] -> w463
              tunnel: w449 -> [w484]
              tunnel: [w482] -> w464
              tunnel: w440 -> [w478]
              tunnel: w439 -> [w477]
              n169 = Search 1D Array(1D array=w478, element=w481) -> (index of element=w480:i32)  [unwired: 1 in]
              n170 = Index Array(array=w477, index=w480) -> (element=w479:string)
              n171 = call-poly <vilib>:"Word Find & Replace.vi"("report in"=w485, "find what?"=w481, "replace with"=w479, "error in (no error)"=w484) -> ("report out"=w483:refnum<class "NI_report.lvclass">, "error out"=w482:errorcluster)  [unwired: 9 in, 1 out]
            }
            n172 = property on="print_calibration" class="Bool (严格)"("DisabledEnum"=T1."Disabled and Grayed Out" ("禁用")) -> ()  [unwired: 2 in, 2 out]
            n173 = call-dynamic "Print Report.vi"("report in"=w463, "error in (no error)"=w464) -> ("report out"=w461:refnum<class "NI_report.lvclass">, "error out"=w462:errorcluster)  [unwired: 12 in]
            n174 = property on="数据写入成功" class="Bool (严格)"("Val(Sgnl)"=FALSE) -> ()  [unwired: 2 in, 2 out]
            n175 = call-dynamic "Dispose Report.vi"("report in"=w461, "error in (no error)"=w462) -> ("error out"=w458:errorcluster)  [unwired: 13 in]
          }
        }
      }
      event "停止": Mouse Up {
        w487 = FALSE
        w489 = T1."Disabled and Grayed Out" ("禁用")
        n176 = event-data() -> ()  [unwired: 1 in, 1 out]
        n177 = property on="init" class="Bool (严格)"("Visible"=TRUE) -> ()  [unwired: 2 in, 2 out]
        n178 = property on="print_calibration" class="Bool (严格)"("DisabledEnum"=w489, "Visible"=w487) -> ()  [unwired: 2 in, 2 out]
        n179 = property on="print_data" class="Bool (严格)"("DisabledEnum"=w489, "Visible"=w487) -> ()  [unwired: 2 in, 2 out]
        n180 = property on="执行状态" class="Bool (严格)"("Val(Sgnl)"=w487) -> ()  [unwired: 2 in, 2 out]
        n181 = local write "初始化成功"(w487) -> ()
        n182 = property on="write" class="Bool (严格)"("Visible"=w487) -> ()  [unwired: 2 in, 2 out]
        n183 = property on="数据写入成功" class="Bool (严格)"("Val(Sgnl)"=w487) -> ()  [unwired: 2 in, 2 out]
      }
    }
    "error out" <- w17
    "执行状态" <- TRUE
  }
  n184 = property on="write" class="Bool (严格)"("Visible"=w8) -> ()  [unwired: 2 in, 2 out]
  n185 = property on="print_calibration" class="Bool (严格)"("DisabledEnum"=w12, "Visible"=w8) -> ()  [unwired: 2 in, 2 out]
  n186 = property on="init" class="Bool (严格)"("Visible"=TRUE) -> ()  [unwired: 2 in, 2 out]
  n187 = property on="print_data" class="Bool (严格)"("DisabledEnum"=w12, "Visible"=w8) -> ()  [unwired: 2 in, 2 out]
